vi "06 Shift Registers.vi"() -> ()   [LabVIEW 2019]
uses:
  _Subs/OpenDiagram/Open_XControl.xctl
panel:
  in  "OpenDiag":refnum<vi>(xcontrol)
  out "n!":i32=120
  in  "n":i32=5
  # "06 Shift Registers\nThis code demonstrates how shift registers work. \n\nA shift register is a way of storing data, structured similarly to an array. With \neach iteration, data in the nth position is moved to the n+1th position. This \nallows you to feed in new data sequentially and access the data of the previous \niteration. \n\nInstructions:\n1. Select Highlight Execution (light bulb on diagram)\n2. Hit run and watch the values on the wires in the block diagram change"
  # "Number of times \nwe run our loop:"
  # "Final generated output:"
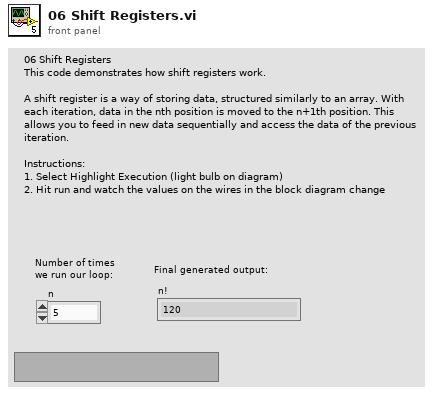
[diagram p1: front panel]
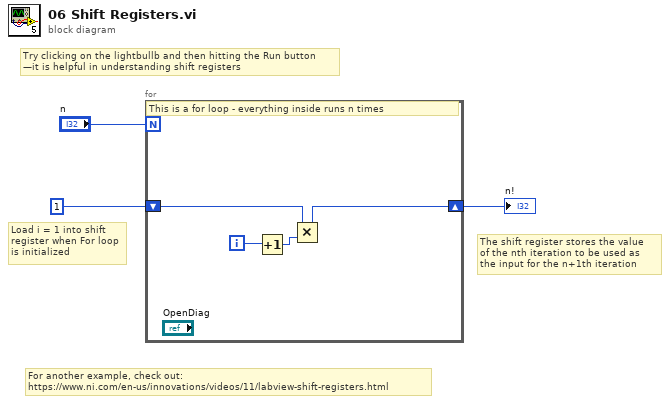
[diagram p0: block diagram]
diagram:
  # "The shift register stores the value \nof the nth iteration to be used as \nthe input for the n+1th iteration"
  # "For another example, check out: \nhttps://www.ni.com/en-us/innovations/videos/11/labview-shift-registers.html"
  # "Load i = 1 into shift register when For loop is initialized"
  # "Try clicking on the lightbullb and then hitting the Run button\n—it is helpful in understanding shift registers"
  n1 = for {
    N: "n" -> [_]
    shift-right: [w4] -> w1
    shift-left: 1 -> [w5]
    i -> [w7]
    # "This is a for loop - everything inside runs n times"
    n2 = Increment(x=w7) -> (x+1=w6:i32)
    n3 = Multiply(x=w5, y=w6) -> (x*y=w4:i32)
  }
  "n!" <- w1
